vi "SS2 Live_Gate Configuration Storage.vi"(7 "Preset Configuration Refnum":refnum<vi>, 8 "Error In":errorcluster, 9 "Action":T1, 10 "Gate Configuration Definition in":T2, 11 "Gate Configuration Name in":string) -> (0 "Error Out":errorcluster, 1 "Configuration ID":i32, 2 "Gate Configuration Definition out":T2, 3 "Gate Configuration Name out":string, 4 "Gate Configuration Found?":bool, 5 "Gate Definition Found?":bool)   [LabVIEW 2019]
uses:
  SS2 Gate Configuration.ctl
  SS2 Gate Definition.ctl
  SS2 Live_Gate Configuration Action.ctl
  <vilib>/UserTags/UserTags.lvlib
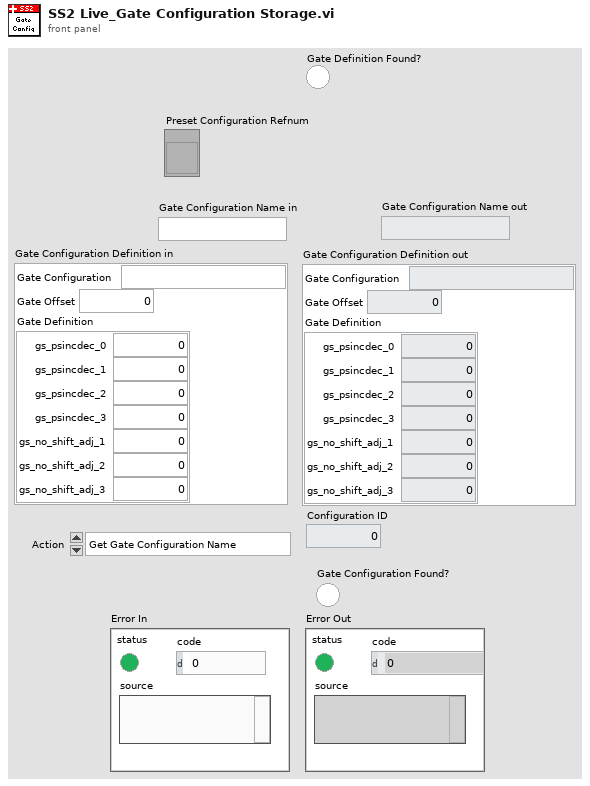
[diagram p1: front panel]
types:
  T1 = typedef "SS2 Live_Gate Configuration Action.ctl" = enum16{"Get Gate Configuration Name", "Get Configuration by Name", "Add Gate Configuration", "Delete Gate Configuration", "Rename Gate Configuration"}
  T2 = typedef "SS2 Gate Configuration.ctl" = cluster{"Gate Configuration":string, "Gate Offset":u32, "Gate Definition":T3}
  T3 = typedef "SS2 Gate Definition.ctl" = cluster{"gs_psincdec_0":u32, "gs_psincdec_1":u32, "gs_psincdec_2":u32, "gs_psincdec_3":u32, "gs_no_shift_adj_1":u32, "gs_no_shift_adj_2":u32, "gs_no_shift_adj_3":u32}
  T4 = enum16{"Left Button", "Center Button", "Right Button", "Window Close"}
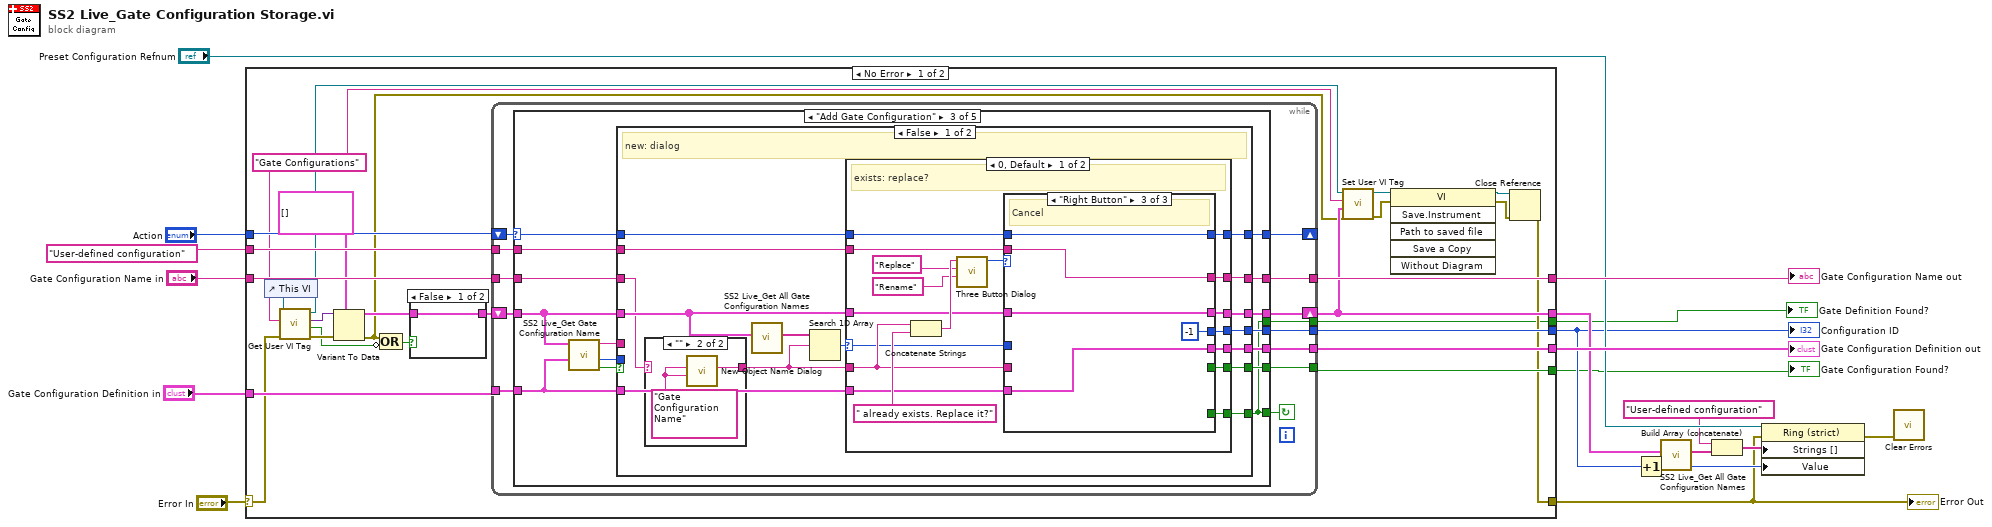
[diagram p0: block diagram]
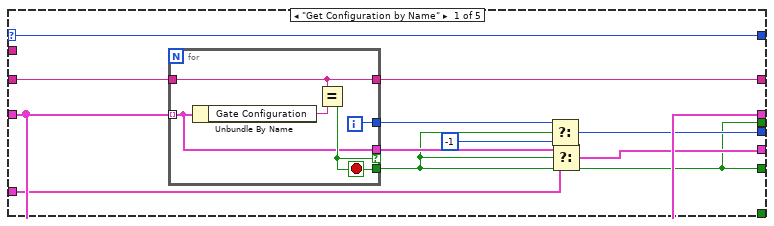
[diagram p3: hidden frame]
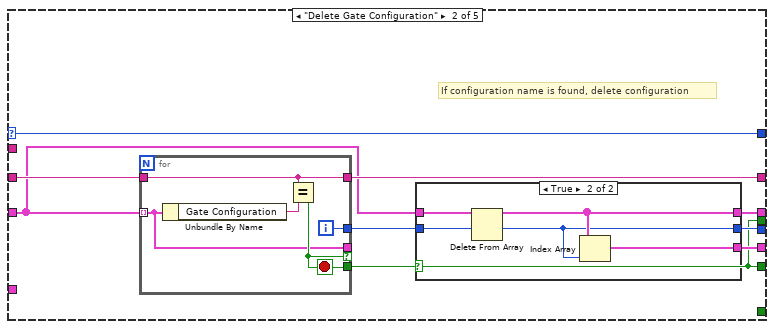
[diagram p4: hidden frame]
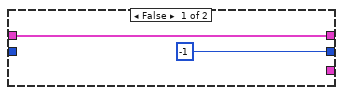
[diagram p5: hidden frame]
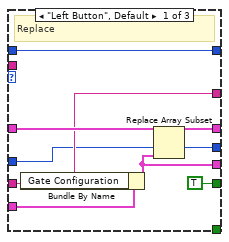
[diagram p7: hidden frame]
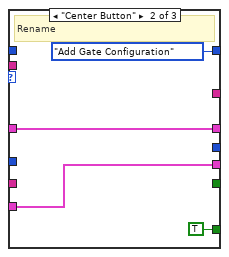
[diagram p8: hidden frame]
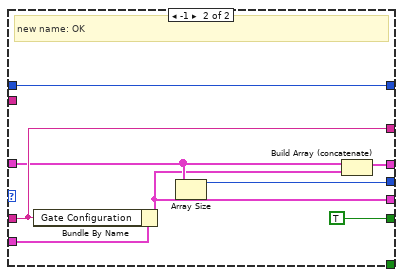
[diagram p9: hidden frame]
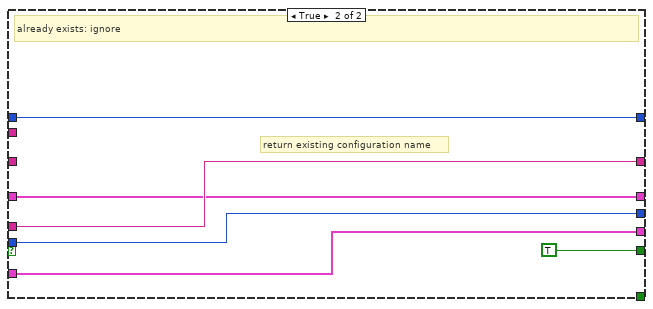
[diagram p10: hidden frame]
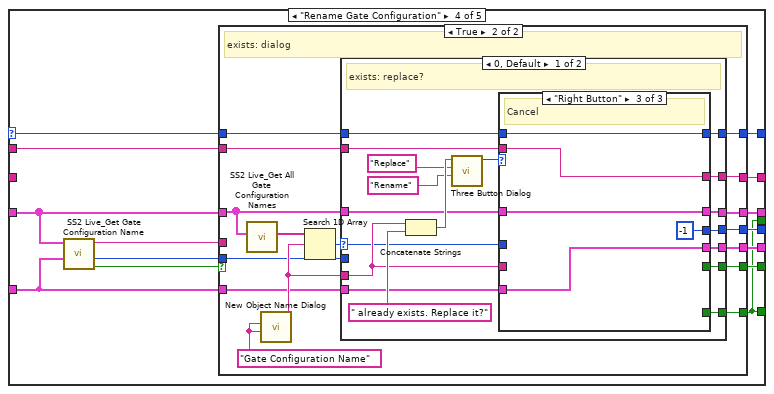
[diagram p11: hidden frame]
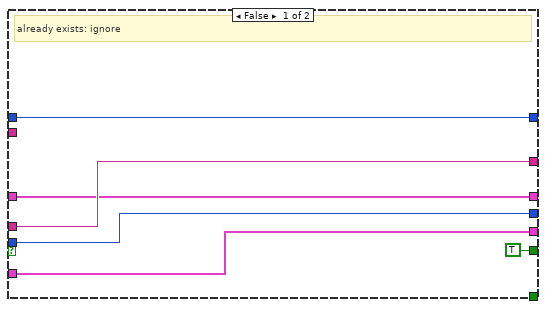
[diagram p12: hidden frame]
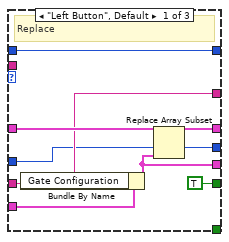
[diagram p13: hidden frame]
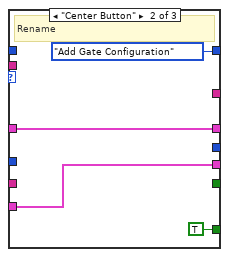
[diagram p14: hidden frame]
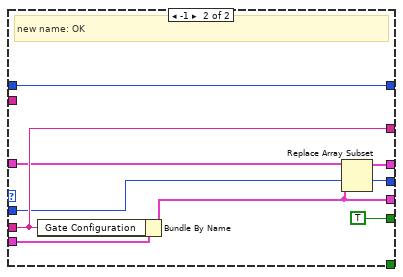
[diagram p15: hidden frame]
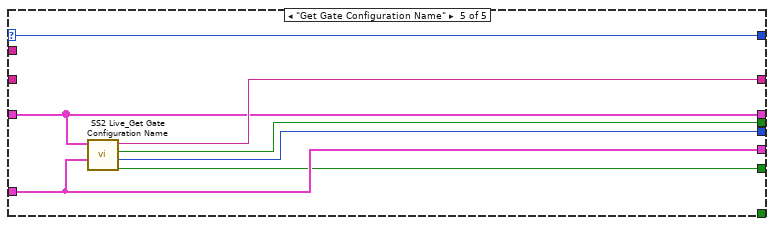
[diagram p16: hidden frame]
diagram:
  n1 = case shown="No Error" "Error In" {
    selector: "Error In" -> [w22 w264]
    tunnel: "Action" -> [w45 _]
    tunnel: "Gate Configuration Name in" -> [w44 _]
    tunnel: [w43 _] -> w16
    tunnel: [w42 _] -> w15
    tunnel: "Gate Configuration Definition in" -> [w41 _]
    tunnel: [w40 _] -> w9
    tunnel: [w39 _] -> w10
    tunnel: "User-defined configuration" ("Object Name out") -> [w38 _]
    tunnel: [w31 _] -> w11
    tunnel: [w20 w264] -> w2
    tunnel: [w19 _] -> w3
    frame No Error {
      w29 = "Gate Configurations" ("Tag Name")
      n2 = control-ref of="This VI"() -> (w37:refnum<vi>)
      n3 = call <vilib>:"Get User VI Tag.vi"("error in (no error)"=w22, "Tag Name"=w29, "VI Refnum"=w37) -> ("error out"=w36:errorcluster, "Was Tag Found?"=w27:bool, "Value"=w35:variant, "dup VI Refnum"=w30:refnum<vi>)  [unwired: 5 in]
      n4 = Variant To Data(error in=w36, type=T2[] [] ("Array"), Variant=w35) -> (data=w33:T2[], error out=w21:errorcluster)
      n5 = Compound Arithmetic op=OR(w21, invert w27) -> (w28:bool)
      n6 = case shown="False" w28 {
        tunnel: w33 -> [w46 _]
        tunnel: [w46 _] -> w32
        frame False {
        }
        frame True {
        }
      }
      n7 = while {
        tunnel: w44 -> [w58]
        shift-right: [w53] -> w31
        shift-left: w32 -> [w57]
        tunnel: [w56] -> w40
        tunnel: [w55] -> w43
        tunnel: [w54] -> w42
        tunnel: w41 -> [w52]
        tunnel: [w51] -> w39
        shift-right: [w50] -> _
        shift-left: w45 -> [w59]
        tunnel: w38 -> [w48]
        tunnel: [w47] -> w19
        stop <- w49 continue-if-true
        n8 = case shown="\"Add Gate Configuration\"" w59 {
          selector: w59 -> [w64 w79 w100 w181 w258]
          tunnel: w58 -> [w70 w84 w97 _ _]
          tunnel: w57 -> [w68 w81 w107 w188 w262]
          tunnel: [w60 w76 w101 w182 w260] -> w56
          tunnel: [w61 w77 w104 w185 w261] -> w55
          tunnel: [w69 w83 w108 w189 w263] -> w54
          tunnel: [w68 w80 w106 w187 w262] -> w53
          tunnel: w52 -> [w62 _ w105 w186 w261]
          tunnel: [w66 w78 w102 w183 w259] -> w51
          tunnel: [w64 w79 w99 w180 w258] -> w50
          tunnel: [_ _ w96 w178 _] -> w49
          tunnel: w48 -> [_ _ w98 w179 _]
          tunnel: [w60 w76 w96 w178 w257] -> w47
          frame "Get Configuration by Name" {
            n9 = for {
              tunnel: w68 -> [w72] mode=indexing
              tunnel: [w74] -> w60
              tunnel: w70 -> [w73]
              tunnel: [w72] -> w63 if=w74
              tunnel: [w73] -> w69
              tunnel: [w71] -> w67
              i -> [w71]
              stop <- w74 stop-if-true
              n10 = Unbundle By Name(w72) -> ("Gate Configuration"=w75:string)
              n11 = Equal?(x=w73, y=w75) -> (x = y?=w74:bool)
            }
            n12 = Select(t=w67, s=w60, f=-1) -> (s? t:f=w66:i32)
            n13 = Select(t=w63, s=w60, f=w62) -> (s? t:f=w61:T2)
          }
          frame "Delete Gate Configuration" {
            # "If configuration name is found, delete configuration"
            n14 = for {
              tunnel: w81 -> [w92] mode=indexing
              tunnel: [w94] -> w76
              tunnel: w84 -> [w93]
              tunnel: [w92] -> _ if=w94
              tunnel: [w93] -> w83
              tunnel: [w91] -> w82
              i -> [w91]
              stop <- w94 stop-if-true
              n15 = Unbundle By Name(w92) -> ("Gate Configuration"=w95:string)
              n16 = Equal?(x=w93, y=w95) -> (x = y?=w94:bool)
            }
            n17 = case shown="True" w76 {
              tunnel: w82 -> [_ w88]
              tunnel: w81 -> [w86 w90]
              tunnel: [w86 w89] -> w80
              tunnel: [-1 w88] -> w78
              tunnel: [_ w87] -> w77
              frame False {
              }
              frame True {
                n18 = Delete From Array(array=w90, index=w88) -> (array with subset deleted=w89:T2[])  [unwired: 1 in, 1 out]
                n19 = Index Array(array=w89, index=w88) -> (element=w87:T2)
              }
            }
          }
          frame "Add Gate Configuration" {
            n20 = call "SS2 Live_Get Gate Configuration Name.vi"("Gate Configuration Definition in"=w105, "Gate Configurations Definitions"=w107) -> ("Gate Configuration Found?"=w110:bool, "Configuration ID"=w103:i32, "Gate Configuration Name"=w109:string)  [unwired: 6 in, 1 out]
            n21 = case shown="False" w110 {
              tunnel: w109 -> [_ w177]
              tunnel: [w120 w177] -> w108
              tunnel: w107 -> [w123 w176]
              tunnel: [w119 w176] -> w106
              tunnel: w105 -> [w121 w175]
              tunnel: [w117 w175] -> w104
              tunnel: w103 -> [_ w174]
              tunnel: [w118 w174] -> w102
              tunnel: [w116 TRUE ("Found?")] -> w101
              tunnel: w100 -> [w115 w173]
              tunnel: [w114 w173] -> w99
              tunnel: [w113 _] -> w96
              tunnel: w98 -> [w112 _]
              tunnel: w97 -> [w111 _]
              frame False {
                # "new: dialog"
                n22 = case shown="\"\"" w111 {
                  selector: w111 -> [w126 _]
                  tunnel: [w126 w127] -> w122
                  frame "Name", Default {
                  }
                  frame "" {
                    w128 = "Gate Configuration Name" ("Object Name in")
                    n23 = call "New Object Name Dialog.vi"("String Name (\"object\")"=w128, "Object Name in"=w128) -> ("Object Name out"=w127:string)  [unwired: 7 in, 2 out]
                  }
                }
                n24 = call "SS2 Live_Get All Gate Configuration Names.vi"("Gate Configurations"=w123) -> ("Gate Configuration Names"=w125:string[])  [unwired: 10 in]
                n25 = Search 1D Array(1D array=w125, element=w122) -> (index of element=w124:i32)  [unwired: 1 in]
                n26 = case shown="0, Default" w124 {
                  selector: w124 -> [w134 _]
                  tunnel: w123 -> [w141 w168]
                  tunnel: w122 -> [w137 w170]
                  tunnel: w121 -> [w130 w171]
                  tunnel: [w136 w170] -> w120
                  tunnel: [w140 w169] -> w119
                  tunnel: [w133 w167] -> w118
                  tunnel: [w129 w166] -> w117
                  tunnel: [w132 TRUE ("Found?")] -> w116
                  tunnel: w115 -> [w139 w165]
                  tunnel: [w138 w165] -> w114
                  tunnel: [w135 _] -> w113
                  tunnel: w112 -> [w131 _]
                  frame 0, Default {
                    # "exists: replace?"
                    n27 = Concatenate Strings(w137, " already exists. Replace it?" ("string")) -> (w145:string)
                    n28 = call <vilib>:"Three Button Dialog.vi"("Center Button Text (\"No\")"="Rename" ("F button name (\"Cancel\")"), "Left Button Text (\"Yes\")"="Replace" ("T button name (\"OK\")"), "message"=w145) -> ("Which Button?"=w142:T4)  [unwired: 8 in]
                    n29 = case shown="\"Right Button\"" w142 {
                      tunnel: w141 -> [w153 w157 w163]
                      tunnel: [w150 w157 w163] -> w140
                      tunnel: w139 -> [w151 _ w162]
                      tunnel: [w151 SS2_Live_Gate_Configuration_Action."Add Gate Configuration" ("Action") w162] -> w138
                      tunnel: w130 -> [w154 w155 w159]
                      tunnel: w137 -> [w152 _ _]
                      tunnel: [w152 _ w161] -> w136
                      tunnel: [_ TRUE _] -> w135
                      tunnel: w134 -> [w149 _ _]
                      tunnel: [w149 _ -1 ("index of element")] -> w133
                      tunnel: [TRUE _ _] -> w132
                      tunnel: w131 -> [_ _ w161]
                      tunnel: [w147 w155 w159] -> w129
                      frame "Left Button", Default {
                        # "Replace"
                        n30 = Bundle By Name(cluster=w154, "Gate Configuration"=w152) -> (w147:T2)
                        n31 = Replace Array Subset(array=w153, new element=w147, index=w149) -> (w150:T2[])
                      }
                      frame "Center Button" {
                        # "Rename"
                      }
                      frame "Right Button" {
                        # "Cancel"
                      }
                    }
                  }
                  frame -1 {
                    # "new name: OK"
                    n32 = Bundle By Name(cluster=w171, "Gate Configuration"=w170) -> (w166:T2)
                    n33 = Array Size(array=w168) -> (size(s)=w167:i32)
                    n34 = Build Array (concatenate)(w168, w166) -> (w169:T2[])
                  }
                }
              }
              frame True {
                # "return existing configuration name"
                # "already exists: ignore"
              }
            }
          }
          frame "Rename Gate Configuration" {
            n35 = call "SS2 Live_Get Gate Configuration Name.vi"("Gate Configuration Definition in"=w186, "Gate Configurations Definitions"=w188) -> ("Gate Configuration Found?"=w191:bool, "Configuration ID"=w184:i32, "Gate Configuration Name"=w190:string)  [unwired: 6 in, 1 out]
            n36 = case shown="True" w191 {
              tunnel: w190 -> [w197 _]
              tunnel: [w197 w207] -> w189
              tunnel: w188 -> [w196 w210]
              tunnel: [w196 w206] -> w187
              tunnel: w186 -> [w195 w208]
              tunnel: [w195 w204] -> w185
              tunnel: w184 -> [w194 w198]
              tunnel: [w194 w205] -> w183
              tunnel: [TRUE ("Found?") w203] -> w182
              tunnel: w181 -> [w193 w202]
              tunnel: [w193 w201] -> w180
              tunnel: [_ w200] -> w178
              tunnel: w179 -> [_ w199]
              frame False {
                # "already exists: ignore"
              }
              frame True {
                w213 = "Gate Configuration Name" ("Object Name in")
                # "exists: dialog"
                n37 = call "SS2 Live_Get All Gate Configuration Names.vi"("Gate Configurations"=w210) -> ("Gate Configuration Names"=w212:string[])  [unwired: 10 in]
                n38 = call "New Object Name Dialog.vi"("String Name (\"object\")"=w213, "Object Name in"=w213) -> ("Object Name out"=w209:string)  [unwired: 7 in, 2 out]
                n39 = Search 1D Array(1D array=w212, element=w209) -> (index of element=w211:i32)  [unwired: 1 in]
                n40 = case shown="0, Default" w211 {
                  selector: w211 -> [w218 _]
                  tunnel: w210 -> [w226 w253]
                  tunnel: w209 -> [w221 w255]
                  tunnel: w208 -> [w222 w256]
                  tunnel: [w220 w255] -> w207
                  tunnel: [w225 w254] -> w206
                  tunnel: [w217 w249] -> w205
                  tunnel: [w214 w250] -> w204
                  tunnel: [w216 TRUE ("Found?")] -> w203
                  tunnel: w202 -> [w224 w252]
                  tunnel: [w223 w252] -> w201
                  tunnel: [w219 _] -> w200
                  tunnel: w199 -> [w215 _]
                  tunnel: w198 -> [_ w249]
                  frame 0, Default {
                    # "exists: replace?"
                    n41 = Concatenate Strings(w221, " already exists. Replace it?" ("string")) -> (w230:string)
                    n42 = call <vilib>:"Three Button Dialog.vi"("Center Button Text (\"No\")"="Rename" ("F button name (\"Cancel\")"), "Left Button Text (\"Yes\")"="Replace" ("T button name (\"OK\")"), "message"=w230) -> ("Which Button?"=w227:T4)  [unwired: 8 in]
                    n43 = case shown="\"Right Button\"" w227 {
                      tunnel: w226 -> [w238 w242 w248]
                      tunnel: [w235 w242 w248] -> w225
                      tunnel: w224 -> [w236 _ w247]
                      tunnel: [w236 SS2_Live_Gate_Configuration_Action."Add Gate Configuration" ("Action") w247] -> w223
                      tunnel: w222 -> [w239 w240 w244]
                      tunnel: w221 -> [w237 _ _]
                      tunnel: [w237 _ w246] -> w220
                      tunnel: [_ TRUE _] -> w219
                      tunnel: w218 -> [w234 _ _]
                      tunnel: [w234 _ -1 ("index of element")] -> w217
                      tunnel: [TRUE _ _] -> w216
                      tunnel: w215 -> [_ _ w246]
                      tunnel: [w232 w240 w244] -> w214
                      frame "Left Button", Default {
                        # "Replace"
                        n44 = Bundle By Name(cluster=w239, "Gate Configuration"=w237) -> (w232:T2)
                        n45 = Replace Array Subset(array=w238, new element=w232, index=w234) -> (w235:T2[])
                      }
                      frame "Center Button" {
                        # "Rename"
                      }
                      frame "Right Button" {
                        # "Cancel"
                      }
                    }
                  }
                  frame -1 {
                    # "new name: OK"
                    n46 = Bundle By Name(cluster=w256, "Gate Configuration"=w255) -> (w250:T2)
                    n47 = Replace Array Subset(array=w253, new element=w250, index=w249) -> (w254:T2[])
                  }
                }
              }
            }
          }
          frame "Get Gate Configuration Name" {
            n48 = call "SS2 Live_Get Gate Configuration Name.vi"("Gate Configuration Definition in"=w261, "Gate Configurations Definitions"=w262) -> ("Gate Configuration Found?"=w260:bool, "Configuration ID"=w259:i32, "Gate Definition Found?"=w257:bool, "Gate Configuration Name"=w263:string)  [unwired: 6 in]
          }
        }
      }
      n49 = call <vilib>:"Set User VI Tag.vi"("error in (no error)"=w21, "Value"=w31, "Tag Name"=w29, "VI Refnum"=w30) -> ("error out"=w24:errorcluster, "dup VI Refnum"=w26:refnum<vi>)  [unwired: 5 in, 1 out]
      n50 = invoke class="VI" method="Save.Instrument"(reference=w26, error in=w24) -> (reference out=w25:refnum<vi>, error out=w23:errorcluster)  [unwired: 4 in, 4 out]
      n51 = Close Reference(reference=w25, error in (no error)=w23) -> (error out=w20:errorcluster)
    }
    frame Error {
    }
  }
  "Error Out" <- w2
  "Gate Configuration Definition out" <- w16
  "Gate Configuration Name out" <- w15
  "Gate Configuration Found?" <- w9
  "Configuration ID" <- w10
  "Gate Definition Found?" <- w3
  n52 = Increment(x=w10) -> (x+1=w6:i32)
  n53 = call "SS2 Live_Get All Gate Configuration Names.vi"("Gate Configurations"=w11) -> ("Gate Configuration Names"=w7:string[])  [unwired: 10 in]
  n54 = Build Array (concatenate)("User-defined configuration" ("element"), w7) -> (w5:string[])
  n55 = property class="Ring (strict)"(reference="Preset Configuration Refnum", error in=w2, "Strings []"=w5, "Value"=w6) -> (error out=w1:errorcluster)  [unwired: 1 out]
  n56 = call <vilib>:"Clear Errors.vi"("error in (no error)"=w1) -> ()  [unwired: 5 in, 2 out]
